vi "STOP_Motor.vi"(9 "error in (no error)":errorcluster, 10 "TCP Network Connection in":refnum<k5>) -> (1 "error out":errorcluster, 2 "TCP Network Connection out":refnum<k5>)   [LabVIEW 2019]
panel:
  out "Command Status":bool
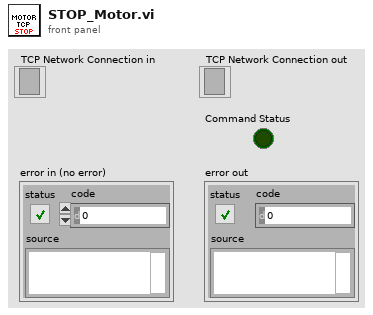
[diagram p1: front panel]
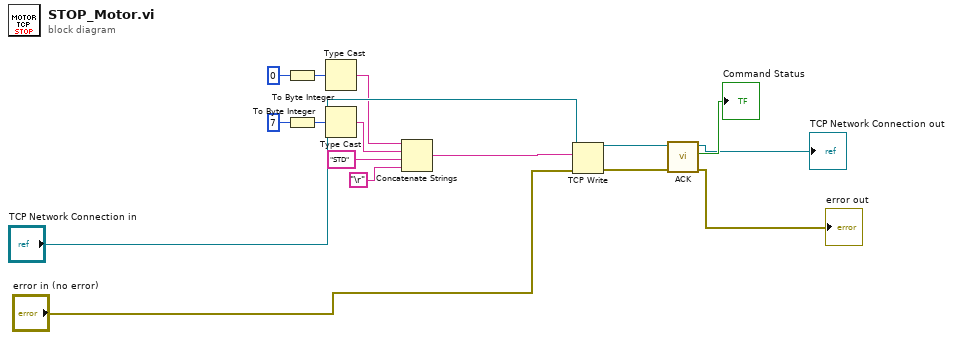
[diagram p0: block diagram]
diagram:
  n1 = To Byte Integer(number=i8 0) -> (8bit integer=w6:i8)
  n2 = To Byte Integer(number=i8 7) -> (8bit integer=w3:i8)
  n3 = Type Cast(x=w6) -> (*(type *) &x=w5:string)  [unwired: 1 in]
  n4 = Type Cast(x=w3) -> (*(type *) &x=w4:string)  [unwired: 1 in]
  n5 = Concatenate Strings(w5, w4, "STD" ("string"), "\r") -> (w9:string)
  n6 = TCP Write(connection ID="TCP Network Connection in", data in=w9, error in (no error)="error in (no error)") -> (connection ID out=w12:refnum<k5>, error out=w13:errorcluster)  [unwired: 1 in, 1 out]
  n7 = call "ACK.vi"("error in (no error)"=w13, "TCP Network Connection in"=w12) -> ("error out"=→"error out":errorcluster, "Command Status"=→"Command Status":bool, "TCP Network Connection out"=→"TCP Network Connection out":refnum<k5>)  [unwired: 7 in]
